vi "通道.vi"() -> (3 "physical channels":tag[](array[tag]))   [LabVIEW 2018]
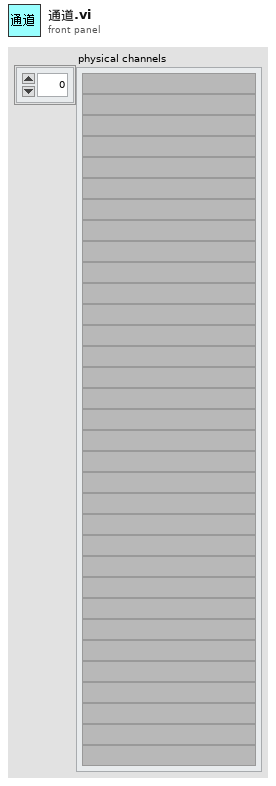
[diagram p1: front panel]
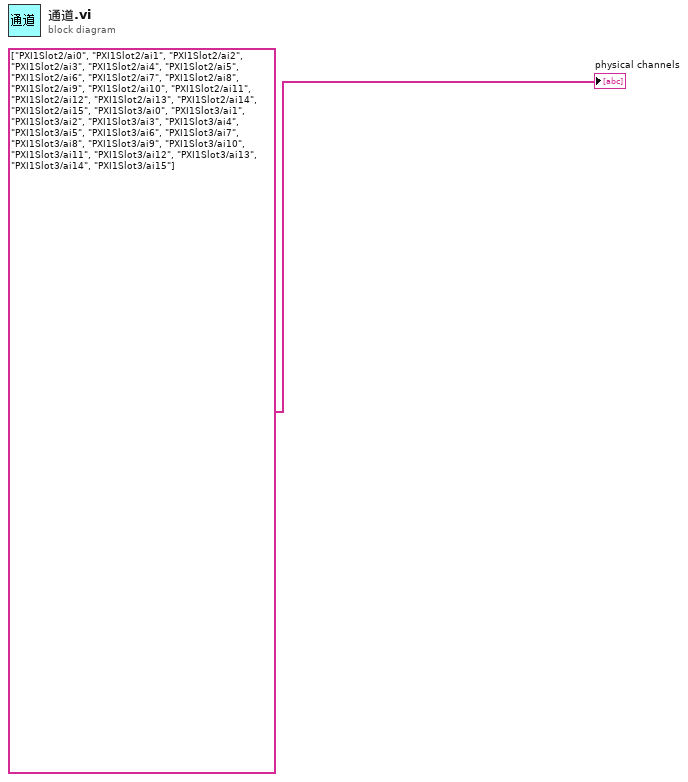
[diagram p0: block diagram]
diagram:
  "physical channels" <- tag[] ["PXI1Slot2/ai0", "PXI1Slot2/ai1", "PXI1Slot2/ai2", "PXI1Slot2/ai3", "PXI1Slot2/ai4", "PXI1Slot2/ai5", "PXI1Slot2/ai6", "PXI1Slot2/ai7", "PXI1Slot2/ai8", "PXI1Slot2/ai9", "PXI1Slot2/ai10", "PXI1Slot2/ai11", "PXI1Slot2/ai12", "PXI1Slot2/ai13", "PXI1Slot2/ai14", "PXI1Slot2/ai15", "PXI1Slot3/ai0", "PXI1Slot3/ai1", "PXI1Slot3/ai2", "PXI1Slot3/ai3", "PXI1Slot3/ai4", "PXI1Slot3/ai5", "PXI1Slot3/ai6", "PXI1Slot3/ai7", "PXI1Slot3/ai8", "PXI1Slot3/ai9", "PXI1Slot3/ai10", "PXI1Slot3/ai11", "PXI1Slot3/ai12", "PXI1Slot3/ai13", "PXI1Slot3/ai14", "PXI1Slot3/ai15"] ("physical channels")
